vi "GV Nmax pixel.vi"() -> ()   [LabVIEW 2017]
panel:
  out "Nmax pixel":u16
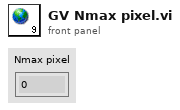
[diagram p1: front panel]
diagram:
